vi "aim and shoot (SubVI).vi"(7 "pin":T1(ring), 8 "error in (no error)":errorcluster, 11 "KNR in":T2) -> (0 "error out":errorcluster, 3 "KNR out":T2)   [LabVIEW 2013]
uses:
  <userlib>/KNR OS 3.0 LabVIEW Toolkit/Type Definition/KNR3 Reference.ctl
  <userlib>/_FPGA Interface Advanced Tools/FPGA Interface Base/FPGA Interface Base.lvclass
  <userlib>/KNR OS 3.0 LabVIEW Toolkit/Type Definition/Resource.ctl
  Global 1.vi
panel:
  out "击球转弯position":i32
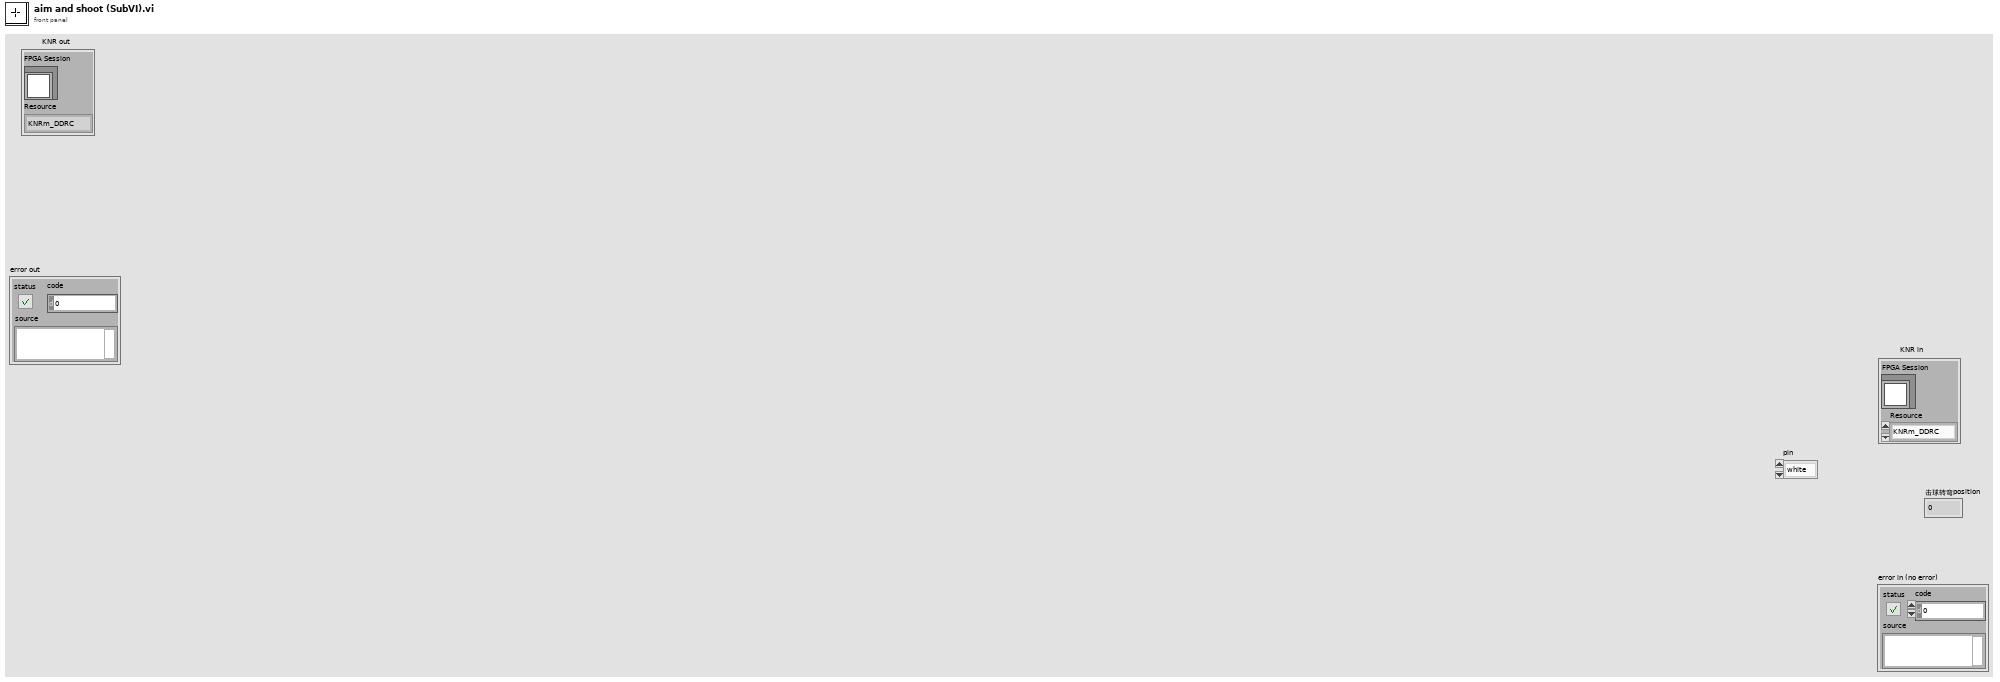
[diagram p1: front panel]
types:
  T1 = enum16{"white", "green", "left", "right", "C1", "C2"}
  T2 = typedef "KNR3 Reference.ctl" = cluster{"FPGA Session":refnum<class "FPGA Interface Base.lvclass">, "Resource":T3}
  T3 = typedef "Resource.ctl" = enum16{"KNRm_DDRC", "KNRm_DDDD", "KNRm_DDDR", "KNRm_DDDC", "KNR"}
  T4 = typedef "DC Motor Port.ctl" = u16
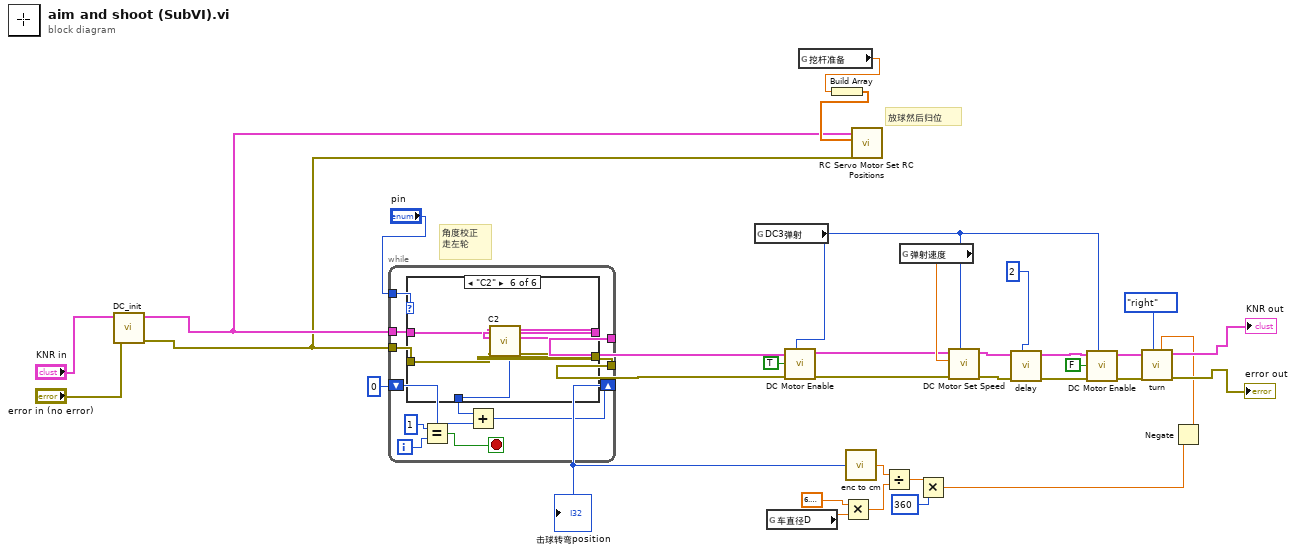
[diagram p0: block diagram]
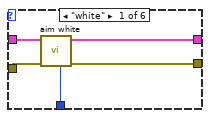
[diagram p2: hidden frame]
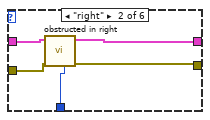
[diagram p3: hidden frame]
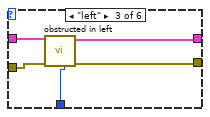
[diagram p4: hidden frame]
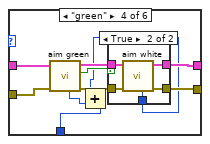
[diagram p5: hidden frame]
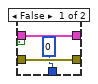
[diagram p6: hidden frame]
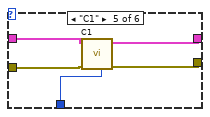
[diagram p7: hidden frame]
diagram:
  # "放球然后归位"
  # "角度校正\n走左轮"
  n1 = call "DC_init.vi"("error in (no error)"="error in (no error)", "KNR in"="KNR in") -> ("error out"=w1:errorcluster, "KNR out"=w2:T2)  [unwired: 6 in, 2 out]
  n2 = while {
    tunnel: w2 -> [w46]
    tunnel: w1 -> [w45]
    tunnel: [w44] -> w4
    tunnel: [w43] -> w3
    shift-right: [w39] -> w32
    shift-left: 0 -> [w37]
    tunnel: "pin" -> [w36]
    i -> [w41]
    stop <- w40 stop-if-true
    n3 = case shown="\"C2\"" w36 {
      tunnel: w46 -> [w51 w55 w60 w71 w84 w89]
      tunnel: w45 -> [w50 w54 w59 w70 w83 w88]
      tunnel: [w49 w53 w58 w68 w82 w87] -> w44
      tunnel: [w48 w52 w57 w67 w81 w86] -> w43
      tunnel: [w47 w56 w61 w62 w80 w85] -> w38
      frame "white" {
        n4 = call "aim white.vi"("error in (no error)"=w50, "KNR in"=w51) -> ("error out"=w48:errorcluster, "KNR out"=w49:T2, "DC Position Offset"=w47:i32)  [unwired: 7 in]
      }
      frame "right" {
        n5 = call "obstructed in right.vi"("error in (no error)"=w54, "KNR in"=w55) -> ("error out"=w52:errorcluster, "KNR out"=w53:T2, "DC Position Offset"=w56:i32)  [unwired: 7 in]
      }
      frame "left" {
        n6 = call "obstructed in left.vi"("error in (no error)"=w59, "KNR in"=w60) -> ("error out"=w57:errorcluster, "KNR out"=w58:T2, "DC Position Offset"=w61:i32)  [unwired: 7 in]
      }
      frame "green" {
        n7 = call "aim green.vi"("error in (no error)"=w70, "KNR in"=w71) -> ("error out"=w66:errorcluster, "Boolean"=w65:bool, "KNR out"=w69:T2, "DC Position Offset"=w63:i32)  [unwired: 6 in]
        n8 = case shown="True" w65 {
          tunnel: w69 -> [w74 w79]
          tunnel: [w74 w78] -> w68
          tunnel: [w73 w77] -> w67
          tunnel: w66 -> [w73 w76]
          tunnel: [0 w75] -> w64
          frame False {
          }
          frame True {
            n9 = call "aim white.vi"("error in (no error)"=w76, "KNR in"=w79) -> ("error out"=w77:errorcluster, "KNR out"=w78:T2, "DC Position Offset"=w75:i32)  [unwired: 7 in]
          }
        }
        n10 = Add(x=w64, y=w63) -> (x+y=w62:i32)
      }
      frame "C1" {
        n11 = call "C1.vi"("error in (no error)"=w83, "KNR in"=w84) -> ("error out"=w81:errorcluster, "KNR out"=w82:T2, "DC Position Offset"=w80:i32)  [unwired: 7 in]
      }
      frame "C2" {
        n12 = call "C2.vi"("error in (no error)"=w88, "KNR in"=w89) -> ("error out"=w86:errorcluster, "KNR out"=w87:T2, "DC Position Offset"=w85:i32)  [unwired: 7 in]
      }
    }
    n13 = Equal?(x=1, y=w41) -> (x = y?=w40:bool)
    n14 = Add(x=w38, y=w37) -> (x+y=w39:i32)
  }
  "击球转弯position" <- w32
  n15 = global read "Global 1.vi" "DC3弹射"() -> (w18:T4)
  n16 = global read "Global 1.vi" "车直径D"() -> (w29:dbl)
  n17 = call <userlib>:"DC Motor Enable.vi"("Port (DS1)"=w18, "error in (no error)"=w3, "Enable Motor(F)"=TRUE, "KNR in"=w4) -> ("error out"=w7:errorcluster, "KNR out"=w8:T2)  [unwired: 6 in]
  n18 = global read "Global 1.vi" "挖杆准备"() -> (w10:dbl)
  n19 = Build Array(w10) -> (w11:dbl[])
  n20 = Multiply(x=6.283185307179586, y=w29) -> (x*y=w28:dbl)
  n21 = call "enc to cm.vi"("E"=w32) -> ("CM"=w31:dbl)  [unwired: 1 in]
  n22 = call <userlib>:"RC Servo Motor Set RC Positions.vi"("error in (no error)"=w1, "RC Pulse Width (1500 uS)"=w11, "KNR in"=w2) -> ()  [unwired: 7 in, 2 out]
  n23 = Divide(x=w31, y=w28) -> (x/y=w27:dbl)
  n24 = global read "Global 1.vi" "弹射速度"() -> (w19:dbl)
  n25 = Multiply(x=w27, y=360) -> (x*y=w22:dbl)
  n26 = call <userlib>:"DC Motor Set Speed.vi"("Port (DS1)"=w18, "error in (no error)"=w7, "Speed (+-100%)"=w19, "KNR in"=w8) -> ("error out"=w16:errorcluster, "KNR out"=w15:T2)  [unwired: 6 in]
  n27 = call "delay.vi"("Numeric"=2, "error in (no error)"=w16, "KNR in"=w15) -> ("error out"=w13:errorcluster, "KNR out"=w14:T2)  [unwired: 7 in]
  n28 = call <userlib>:"DC Motor Enable.vi"("Port (DS1)"=w18, "error in (no error)"=w13, "Enable Motor(F)"=FALSE, "KNR in"=w14) -> ("error out"=w5:errorcluster, "KNR out"=w6:T2)  [unwired: 6 in]
  n29 = Negate(x=w22) -> (-x=w21:dbl)
  n30 = call "turn.vi"("Angle"=w21, "side"=enum16{"right", "left"}."right", "error in (no error)"=w5, "KNR in"=w6) -> ("error out"=→"error out":errorcluster, "KNR out"=→"KNR out":T2)  [unwired: 6 in]
